vi "Bar.vi"(4 "Properties":T1={"Bar Color"=2147483647, "Line"={"Style"=enum."Automatic", "Color"=2147483647, "Width"=nan}, "Display"={"Alpha"=nan, "Z Order"=nan}} {"Line"."Color" items=["Automatic"=2147483647, "Black"=0, "White"=16777215, "Red"=16711680, "Green"=2263842, "Blue"=255, "Cyan"=65535, "Magenta"=16711935, "Yellow"=16776960]; "Bar Color" items=["Automatic"=2147483647, "Black"=0, "White"=16777215, "Red"=16711680, "Green"=2263842, "Blue"=255, "Cyan"=65535, "Magenta"=16711935, "Yellow"=16776960]}, 5 "Bar Bottoms":dbl[](array[numeric]), 6 "Legend Title":string, 7 "Bar Widths":dbl[](array[numeric]), 8 "error in (no error)":errorcluster, 9 "Bar Lengths":dbl[](array[numeric]), 10 "X Coordinates":dbl[](array[numeric]), 11 "Plot ID":T6 format="%x") -> (0 "error out":errorcluster, 3 "Plot ID Out":T6 format="%x")   [LabVIEW 2013, in "Advanced Plotting Toolkit.lvlib"]
doc: "Make a bar plot. The only required input is the bar lengths. You can also specify the X positions of the bar centers (defaults to 0, 1, 2...), widths for the bars, and starting Y locations for the bars (defaults to y=0)."
uses:
  Advanced Plotting Toolkit.lvlib
  typedefs/PlotID.ctl
  BarProperties.ctl
  typedefs/PlotColor.ctl
  properties/Line.ctl
  properties/Line_Style.ctl
  properties/Display.ctl
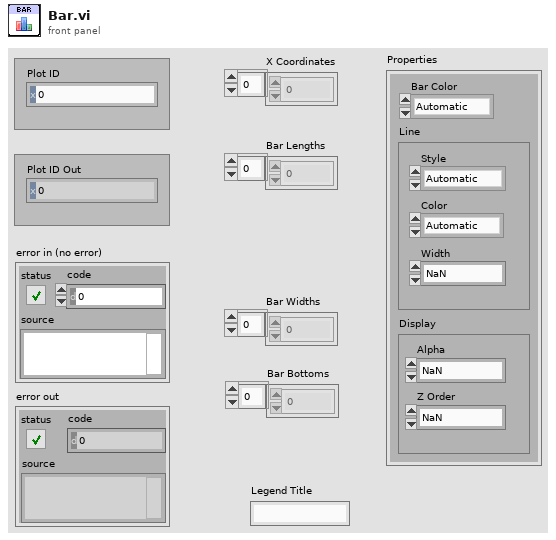
[diagram p1: front panel]
types:
  T1 = typedef "Advanced Plotting Toolkit.lvlib/BarProperties.ctl" = cluster{"Bar Color":T2, "Line":T3, "Display":T5}
  T2 = typedef "Advanced Plotting Toolkit.lvlib/PlotColor.ctl" = u32
  T3 = typedef "Advanced Plotting Toolkit.lvlib/Line.ctl" = cluster{"Style":T4, "Color":T2, "Width":sgl}
  T4 = typedef "Advanced Plotting Toolkit.lvlib/Line_Style.ctl" = enum16{"Automatic", "Solid", "Dashed", "Dotted", "Dash-dot", "Invisible"}
  T5 = typedef "Advanced Plotting Toolkit.lvlib/Display.ctl" = cluster{"Alpha":dbl, "Z Order":dbl}
  T6 = typedef "Advanced Plotting Toolkit.lvlib/PlotID.ctl" = i32
  T7 = typedef "Advanced Plotting Toolkit.lvlib/KeyValue.ctl" = cluster{"Key":string, "Value":string}
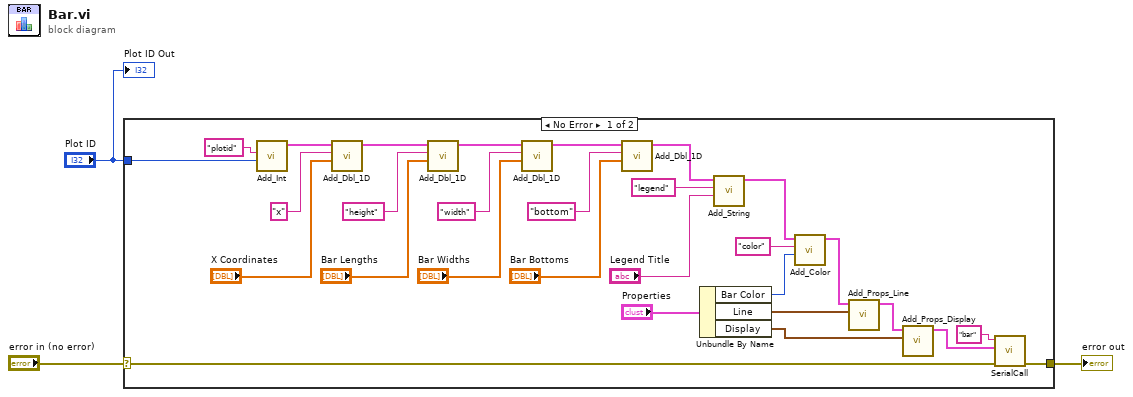
[diagram p0: block diagram]
diagram:
  n1 = case shown="No Error" "error in (no error)" {
    selector: "error in (no error)" -> [w17 w33]
    tunnel: "Plot ID" -> [w32 _]
    tunnel: [w16 w33] -> w1
    frame No Error {
      n2 = call "Add_Int.vi"("Value"=w32, "Key"="plotid") -> ("Keyword Array Out"=w26:T7[])  [unwired: 9 in]
      n3 = call "Add_Dbl_1D.vi"("Value"="X Coordinates", "Key"="x", "Keyword Array"=w26) -> ("Keyword Array Out"=w25:T7[])  [unwired: 8 in]
      n4 = call "Add_Dbl_1D.vi"("Value"="Bar Lengths", "Key"="height", "Keyword Array"=w25) -> ("Keyword Array Out"=w22:T7[])  [unwired: 8 in]
      n5 = call "Add_Dbl_1D.vi"("Value"="Bar Widths", "Key"="width", "Keyword Array"=w22) -> ("Keyword Array Out"=w14:T7[])  [unwired: 8 in]
      n6 = call "Add_Dbl_1D.vi"("Value"="Bar Bottoms", "Key"="bottom", "Keyword Array"=w14) -> ("Keyword Array Out"=w7:T7[])  [unwired: 8 in]
      n7 = Unbundle By Name("Properties") -> ("Bar Color"=w9:T2, "Line"=w11:T3, "Display"=w10:T5)
      n8 = call "Add_String.vi"("Value"="Legend Title", "Key"="legend", "Keyword Array"=w7) -> ("Keyword Array Out"=w6:T7[])  [unwired: 8 in]
      n9 = call "Add_Color.vi"("Color"=w9, "Key"="color", "Keyword Array"=w6) -> ("Keyword Array Out"=w8:T7[])  [unwired: 8 in]
      n10 = call "Add_Props_Line.vi"("Line"=w11, "Keyword Array"=w8) -> ("Keyword Array Out"=w13:T7[])  [unwired: 9 in]
      n11 = call "Add_Props_Display.vi"("Display"=w10, "Keyword Array"=w13) -> ("Keyword Array Out"=w12:T7[])  [unwired: 9 in]
      n12 = call "SerialCall.vi"("error in (no error)"=w17, "data"=w12, "Resource"="bar") -> ("error out"=w16:errorcluster)  [unwired: 7 in, 1 out]
    }
    frame Error {
    }
  }
  "error out" <- w1
  "Plot ID Out" <- "Plot ID"
